vi "Check CRC.vi"(10 "Msg Names CRC":u32, 11 "Group in":refnum<class "Group.lvclass">) -> (2 "CRC Matches":bool, 3 "Group out":refnum<class "Group.lvclass">)   [LabVIEW 2020, in "Vecto.lvlib" / "Group.lvclass"]
uses:
  Group.lvclass
  Group.lvclass/Group.ctl
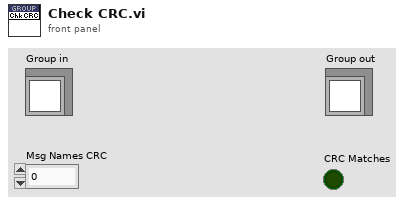
[diagram p1: front panel]
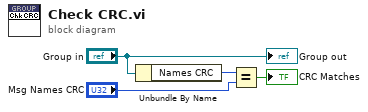
[diagram p0: block diagram]
diagram:
  n1 = Unbundle By Name("Group in") -> ("Names CRC"=w3:u32)
  n2 = Equal?(x=w3, y="Msg Names CRC") -> (x = y?=→"CRC Matches":bool)
  "Group out" <- "Group in"
